vi "创建水质参数数据表.vi"() -> ()   [LabVIEW 2016, in "数据查询.lvlib"]
uses:
  <vilib>/Utility/sysdir.llb/System Directory Type.ctl
  <vilib>/addons/database/Auxilliary.llb/DB Tools Column Info.ctl
  <vilib>/addons/database/Auxilliary.llb/DB Tools DataTypes.ctl
  <vilib>/addons/database/Connection.llb/DB Tools Open Connec (String).vi
  <vilib>/addons/database/NI_Database_API.lvlib
  <vilib>/Utility/VariantDataType/VariantType.lvlib
panel:
  in  "data in":T1
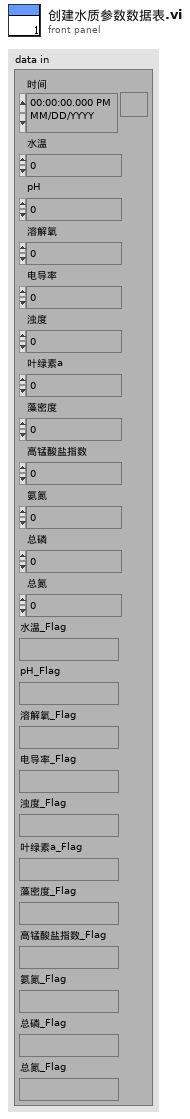
[diagram p1: front panel]
types:
  T1 = cluster{"时间":timestamp, "水温":sgl, "pH":sgl, "溶解氧":sgl, "电导率":sgl, "浊度":sgl, "叶绿素a":sgl, "藻密度":sgl, "高锰酸盐指数":sgl, "氨氮":sgl, "总磷":sgl, "总氮":sgl, "水温_Flag":string, "pH_Flag":string, "溶解氧_Flag":string, "电导率_Flag":string, "浊度_Flag":string, "叶绿素a_Flag":string, "藻密度_Flag":string, "高锰酸盐指数_Flag":string, "氨氮_Flag":string, "总磷_Flag":string, "总氮_Flag":string}
  T2 = typedef "System Directory Type.ctl" = i32
  T3 = typedef "NI_Database_API.lvlib/DB Tools Column Info.ctl" = cluster{"column name":string, "data type":T4, "size":i32, "allow null?":bool}
  T4 = typedef "NI_Database_API.lvlib/DB Tools DataTypes.ctl" = enum16{"String", "Long (I32)", "Single (SGL)", "Double (DBL)", "Date/Time", "Binary"}
  T5 = typedef "VariantType.lvlib/Type.ctl" = enum8{"Invalid Type", "Void", "I8", "I16", "I32", "I64", "U8", "U16", "U32", "U64", "Single Float", "Double Float", "Extended Float", "Single Complex", "Double Complex", "Extended Complex", "Enum U8", "Enum U16", "Enum U32", "Enum U64", "Single Float With Unit", "Double Float With Unit", "Extended Float With Unit", "Single Complex with Unit", "Double Complex with Unit", "Extended Complex with Unit", "Boolean", "String", "Path", "Picture", "Tag", "Array", "Cluster", "Variant", "LV Variant", "Waveform", "Timestamp", "Digital Waveform", "Digital Data", "ExpressData", "Refnum", "External Data", "VI", "Poly VI", "LabVIEW Class Instance", "Fixed Point"}
  T6 = typedef "NI_Database_API.lvlib/Conn ObjectReference.ctl" = refnum<k1>
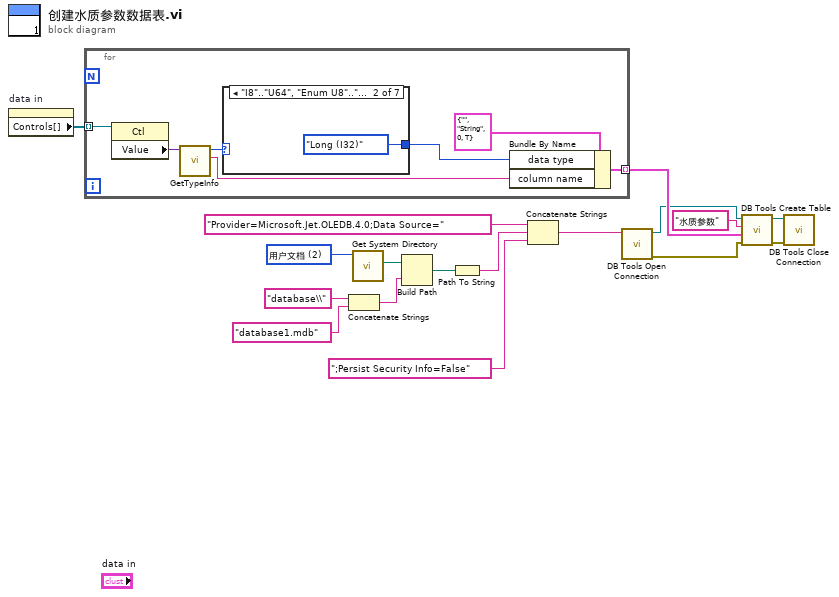
[diagram p0: block diagram]
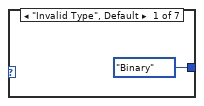
[diagram p2: hidden frame]
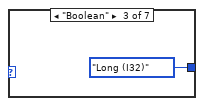
[diagram p3: hidden frame]
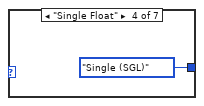
[diagram p4: hidden frame]
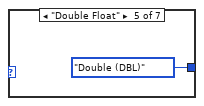
[diagram p5: hidden frame]
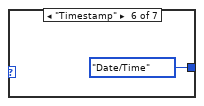
[diagram p6: hidden frame]
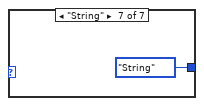
[diagram p7: hidden frame]
diagram:
  w14 = T2 2 items=["用户目录"=0, "用户桌面"=1, "用户文档"=2, "用户应用程序数据"=3, "用户设置"=4, "用户临时目录"=5, "公共文档"=6, "公共应用程序数据"=7, "公共设置"=8, "公共缓存"=13, "系统核心库"=9, "系统安装库"=10, "应用程序文件"=11, "启动盘根目录"=12] ("system directory type")
  n1 = property on="data in" class="Clust (严格)"() -> ("Controls[]"=w17:refnum<vi>[])  [unwired: 2 in, 2 out]
  n2 = for {
    tunnel: w17 -> [w24] mode=indexing
    tunnel: [w20] -> w15 mode=indexing
    n3 = property class="Ctl"(reference=w24) -> ("Value"=w19:variant)  [unwired: 1 in, 2 out]
    n4 = call <vilib>:"GetTypeInfo.vi"("Variant"=w19) -> ("Name"=w18:string, "Type Enum"=w22:T5)  [unwired: 6 in, 3 out]
    n5 = case shown="\"I8\"..\"U64\", \"Enum U8\"..\"Enum U64\"" w22 {
      tunnel: [DB_Tools_DataTypes."Binary" ("data type") DB_Tools_DataTypes."Long (I32)" ("data type") DB_Tools_DataTypes."Long (I32)" ("data type") DB_Tools_DataTypes."Single (SGL)" ("data type") DB_Tools_DataTypes."Double (DBL)" ("data type") DB_Tools_DataTypes."Date/Time" ("data type") DB_Tools_DataTypes."String" ("data type")] -> w21
      frame "Invalid Type", Default {
      }
      frame "I8".."U64", "Enum U8".."Enum U64" {
      }
      frame "Boolean" {
      }
      frame "Single Float" {
      }
      frame "Double Float" {
      }
      frame "Timestamp" {
      }
      frame "String" {
      }
    }
    n6 = Bundle By Name(cluster=T3 {"column name"="", "data type"=enum."String", "size"=0, "allow null?"=TRUE} ("column information"), "data type"=w21, "column name"=w18) -> (w20:T3)
  }
  n7 = Concatenate Strings("database\\" ("condition"), "database1.mdb" ("database")) -> (w6:string)
  n8 = call <vilib>:"Get System Directory.vi"("system directory type"=w14) -> ("system directory"=w12:path)  [unwired: 10 in]
  n9 = Build Path(base path=w12, name or relative path=w6) -> (appended path=w11:path)
  n10 = Path To String(path=w11) -> (string=w10:string)
  n11 = Concatenate Strings("Provider=Microsoft.Jet.OLEDB.4.0;Data Source=" ("condition"), w10, ";Persist Security Info=False" ("condition")) -> (w8:string)
  n12 = call-poly <vilib>:"DB Tools Open Connection.vi"("connection information"=w8) -> ("error out"=w3:errorcluster, "connection reference"=w4:T6)  [unwired: 7 in]
  n13 = call <vilib>:"DB Tools Create Table.vi"("error in (no error)"=w3, "column information"=w15, "table"="水质参数", "connection reference"=w4) -> ("error out"=w2:errorcluster, "connection reference out"=w1:T6)  [unwired: 4 in]
  n14 = call <vilib>:"DB Tools Close Connection.vi"("error in (no error)"=w2, "connection reference"=w1) -> ()  [unwired: 5 in, 1 out]
